vi "Raise Shooter.vi"(8 "error in (no error)":errorcluster) -> (0 "error out":errorcluster)   [LabVIEW 2017]
uses:
  <vilib>/Rock Robotics/WPI/Solenoid/WPI_SolenoidValue.ctl
  <vilib>/Rock Robotics/WPI/Solenoid/WPI_SolenoidSetEnum.vi
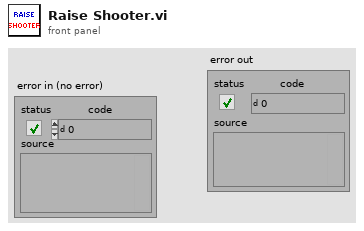
[diagram p1: front panel]
types:
  T1 = typedef "WPI_SolenoidValue.ctl" = enum16{"Off", "On", "Forward", "Reverse"}
  T2 = typedef "WPI_SolenoidDevRef.ctl" = cluster{"DevStatus":errorcluster, "Pneumatics Control Module":u8, "Forward Solenoid Channel":T3, "Reverse Solenoid Channel":T3}
  T3 = typedef "WPI_SolenoidChannel.ctl" = enum8{"Solenoid 0", "Solenoid 1", "Solenoid 2", "Solenoid 3", "Solenoid 4", "Solenoid 5", "Solenoid 6", "Solenoid 7", "Invalid"}
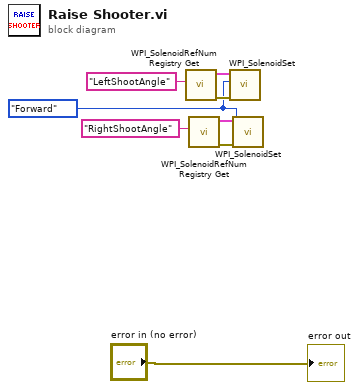
[diagram p0: block diagram]
diagram:
  w1 = WPI_SolenoidValue."Forward" ("Value")
  n1 = call <vilib>:"WPI_SolenoidRefNum Registry Get.vi"("refnum name"="LeftShootAngle") -> ("error out"=w7:errorcluster, "SolenoidDevRef"=w6:T2)  [unwired: 9 in]
  n2 = call <vilib>:"WPI_SolenoidRefNum Registry Get.vi"("refnum name"="RightShootAngle") -> ("error out"=w2:errorcluster, "SolenoidDevRef"=w3:T2)  [unwired: 9 in]
  n3 = call-poly <vilib>:"WPI_SolenoidSet.vi"("error in (no error)"=w7, "Value"=w1, "SolenoidDevRef"=w6) -> ()  [unwired: 7 in, 2 out]
  n4 = call-poly <vilib>:"WPI_SolenoidSet.vi"("error in (no error)"=w2, "Value"=w1, "SolenoidDevRef"=w3) -> ()  [unwired: 7 in, 2 out]
  "error out" <- "error in (no error)"
